vi "Write SSH Client.vi"(8 "error in (no error)":errorcluster, 10 "NI_SSH.lvlib:SSH Client":refnum<class "Generic Client.lvclass">, 11 "session in":refnum<class "Session.lvclass">) -> (0 "error out":errorcluster, 3 "session out":refnum<class "Session.lvclass">)   [LabVIEW 2020, in "NI_SFTP.lvlib" / "Session.lvclass"]
uses:
  <vilib>/net/SFTP/Session/Session.lvclass
  <vilib>/net/SSH/Client/Generic/Generic Client.lvclass
  <vilib>/net/SFTP/Session/Session.lvclass/Session.ctl
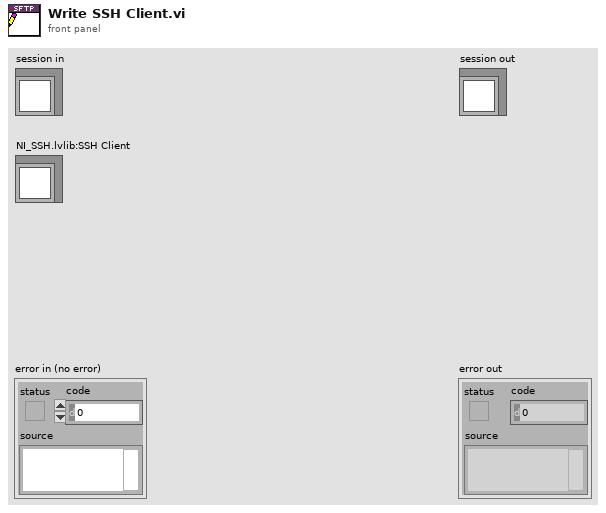
[diagram p1: front panel]
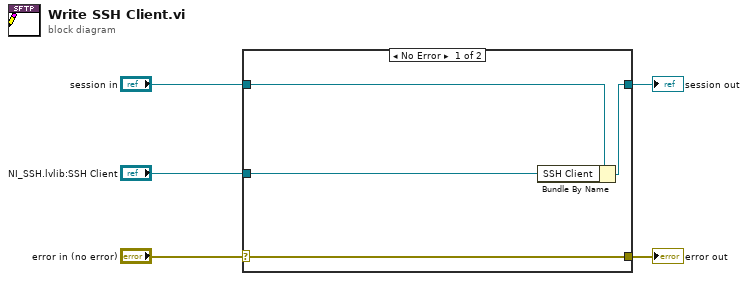
[diagram p0: block diagram]
diagram:
  n1 = case shown="No Error" "error in (no error)" {
    selector: "error in (no error)" -> [w9 w10]
    tunnel: [w9 w10] -> w4
    tunnel: [w7 w11] -> w2
    tunnel: "session in" -> [w8 w11]
    tunnel: "NI_SSH.lvlib:SSH Client" -> [w6 _]
    frame No Error {
      n2 = Bundle By Name(cluster=w8, "SSH Client"=w6) -> (w7:refnum<class "Session.lvclass">)
    }
    frame Error {
    }
  }
  "error out" <- w4
  "session out" <- w2
